vi "New Test Window Launched.vi"(8 "error in (no error)":errorcluster, 9 "VI Refnum":refnum<vi>, 10 "Window Name":string, 11 "Test Application Controller in":refnum<class "Test Application Controller.lvclass">) -> (0 "error out":errorcluster, 3 "Test Application Controller out":refnum<class "Test Application Controller.lvclass">)   [LabVIEW 2017, in "Test Application Controller.lvlib" / "Test Application Controller.lvclass"]
uses:
  Test Application Controller.lvclass
  Test Application Controller.lvclass/Test Application Controller.ctl
  User Interface Messages/Update SubPanel Msg/Update SubPanel Msg.lvclass/Update SubPanel Msg.ctl
  <vilib>/ActorFramework/Message Enqueuer/Message Enqueuer.lvclass/Message Enqueuer.ctl
  <vilib>/ActorFramework/Message Enqueuer/Enqueue.vi
  User Interface Messages/Update SubPanel Msg/Update SubPanel Msg.lvclass
  C:/Program Files (x86)/National Instruments/LabVIEW 2017/vi.lib/ActorFramework/Message/Message.lvclass
  <vilib>/ActorFramework/Message Priority Queue/Priority Enqueue.vi
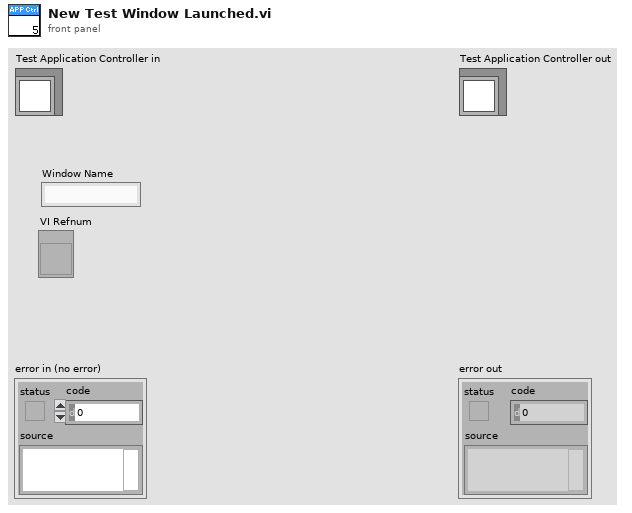
[diagram p1: front panel]
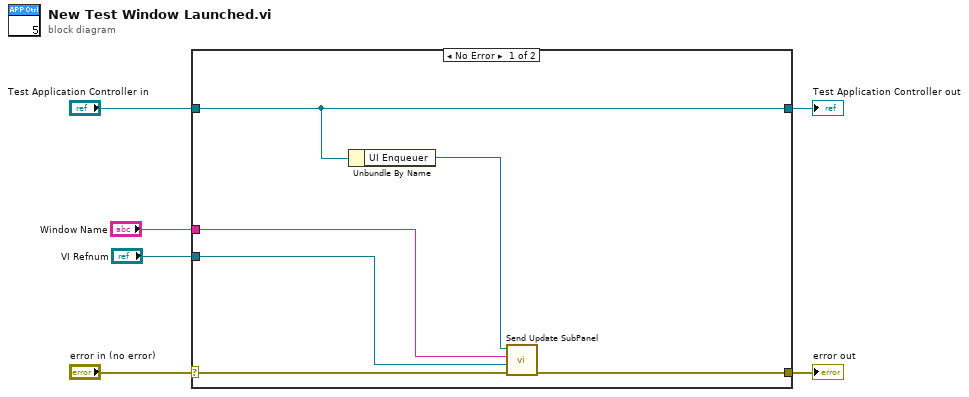
[diagram p0: block diagram]
diagram:
  n1 = case shown="No Error" "error in (no error)" {
    selector: "error in (no error)" -> [w11 w14]
    tunnel: [w10 w14] -> w5
    tunnel: [w12 w13] -> w3
    tunnel: "Test Application Controller in" -> [w12 w13]
    tunnel: "Window Name" -> [w8 _]
    tunnel: "VI Refnum" -> [w7 _]
    frame No Error {
      n2 = Unbundle By Name(w12) -> ("UI Enqueuer"=w9:refnum<class "Message Enqueuer.lvclass">)
      n3 = call "Send Update SubPanel.vi"("error in (no error)"=w11, "VI Refnum"=w7, "Window Name"=w8, "Message Enqueuer"=w9) -> ("error out"=w10:errorcluster)  [unwired: 6 in, 1 out]
    }
    frame Error {
    }
  }
  "error out" <- w5
  "Test Application Controller out" <- w3
